vi "kloehn V6 - Parse Pesponse.vi"(8 "error in":errorcluster, 11 "Response String":string) -> (0 "error out":errorcluster, 2 "Status":enum16{"Ready", "Busy"}(ring), 3 "Response String":string)   [LabVIEW 2010]
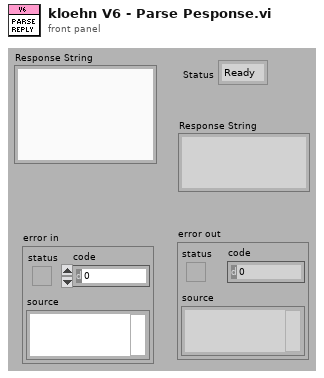
[diagram p1: front panel]
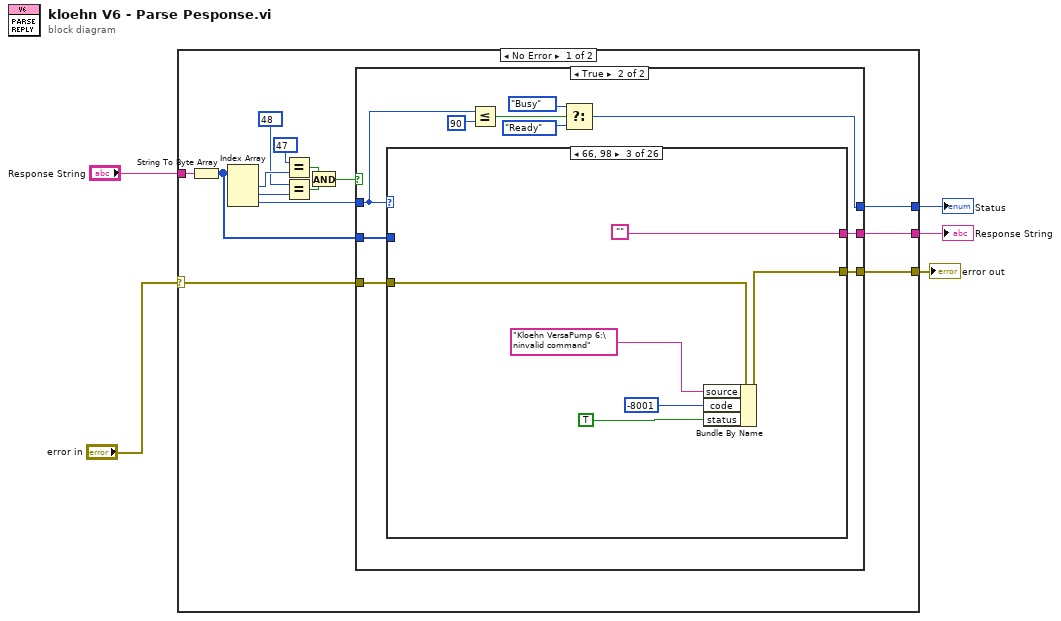
[diagram p0: block diagram]
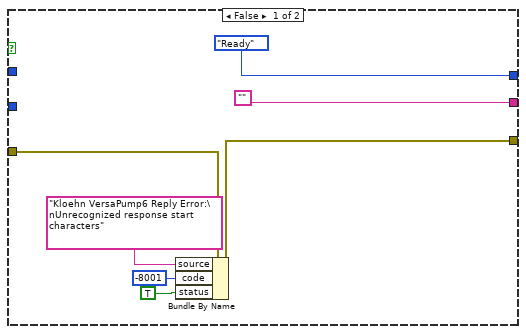
[diagram p2: hidden frame]
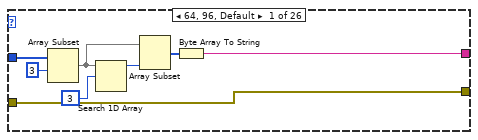
[diagram p3: hidden frame]
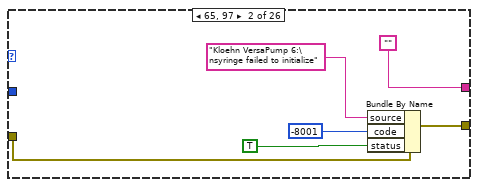
[diagram p4: hidden frame]
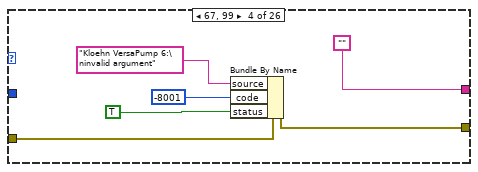
[diagram p5: hidden frame]
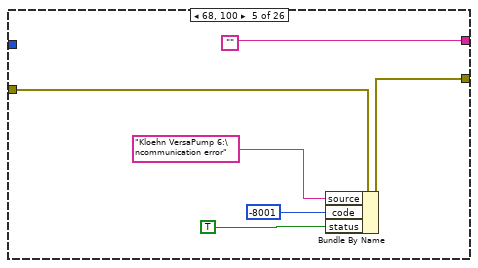
[diagram p6: hidden frame]
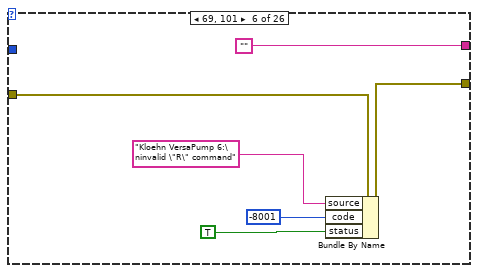
[diagram p7: hidden frame]
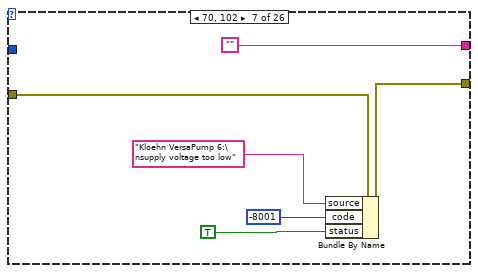
[diagram p8: hidden frame]
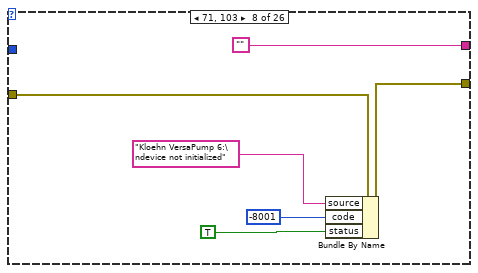
[diagram p9: hidden frame]
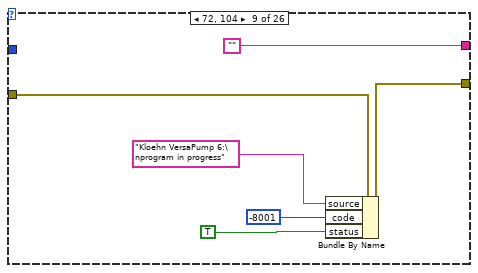
[diagram p10: hidden frame]
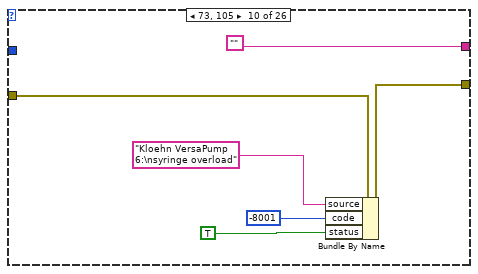
[diagram p11: hidden frame]
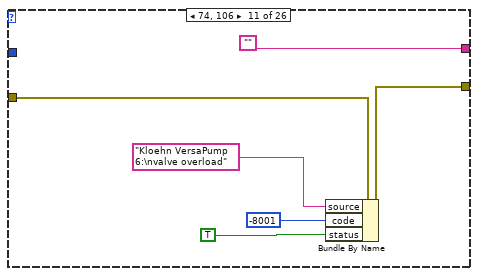
[diagram p12: hidden frame]
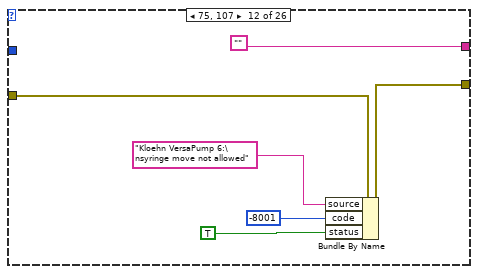
[diagram p13: hidden frame]
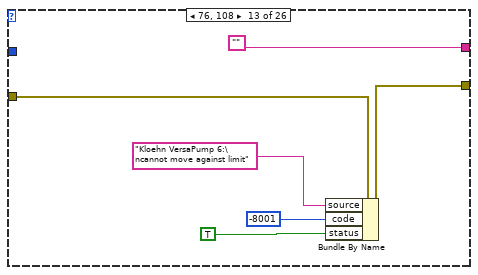
[diagram p14: hidden frame]
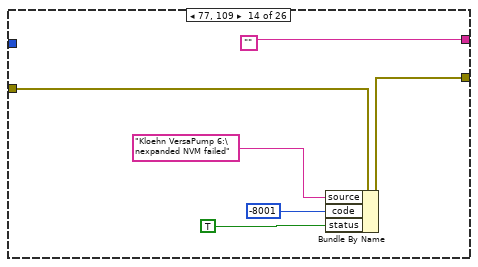
[diagram p15: hidden frame]
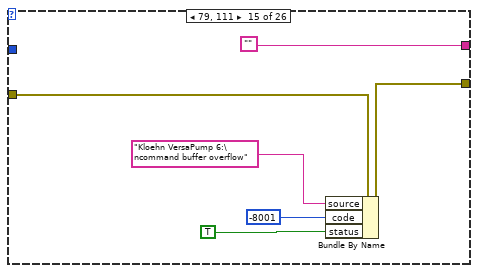
[diagram p16: hidden frame]
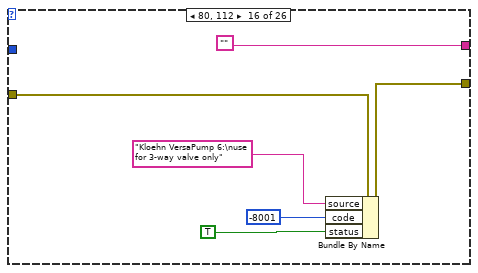
[diagram p17: hidden frame]
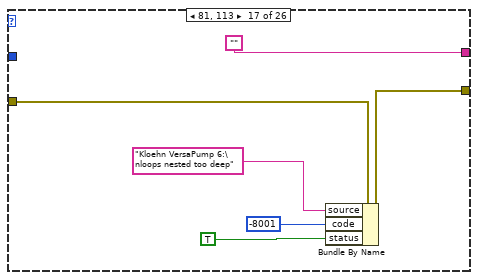
[diagram p18: hidden frame]
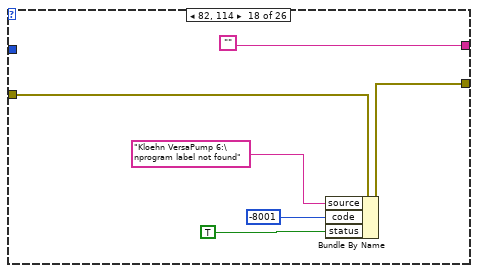
[diagram p19: hidden frame]
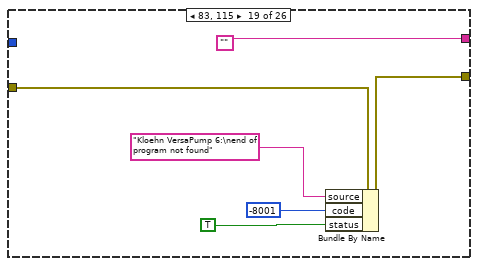
[diagram p20: hidden frame]
diagram:
  n1 = case shown="No Error" "error in" {
    selector: "error in" -> [w11 w197]
    tunnel: "Response String" -> [w19 _]
    tunnel: [w10 w197] -> w3
    tunnel: [w8 enum16{"Ready", "Busy"}."Busy" ("Status")] -> w2
    tunnel: [w6 ""] -> w1
    frame No Error {
      n2 = String To Byte Array(string=w19) -> (unsigned byte array=w7:u8[])
      n3 = Index Array(array=w7) -> (element #1=w18:u8, element #2=w16:u8, element #3=w9:u8)  [unwired: 3 in]
      n4 = Equal?(x=u8 47, y=w18) -> (x = y?=w14:bool)
      n5 = Equal?(x=u8 48, y=w16) -> (x = y?=w13:bool)
      n6 = And(x=w14, y=w13) -> (x .and. y?=w12:bool)
      n7 = case shown="True" w12 {
        tunnel: w11 -> [w26 w36]
        tunnel: [w25 w35] -> w10
        tunnel: w9 -> [_ w30]
        tunnel: [enum16{"Ready", "Busy"}."Ready" ("Status") w29] -> w8
        tunnel: w7 -> [_ w28]
        tunnel: ["" w27] -> w6
        frame False {
          n8 = Bundle By Name(cluster=w26, "source"="Kloehn VersaPump6 Reply Error:\nUnrecognized response start characters", "code"=-8001, "status"=TRUE) -> (w25:errorcluster)
        }
        frame True {
          n9 = case shown="66, 98" w30 {
            tunnel: w36 -> [w44 w50 w56 w62 w68 w74 w80 w86 w92 w98 w104 w110 w116 w122 w128 w134 w140 w146 w152 w158 w164 w170 w176 w182 w188 w194]
            tunnel: [w44 w49 w55 w61 w67 w73 w79 w85 w91 w97 w103 w109 w115 w121 w127 w133 w139 w145 w151 w157 w163 w169 w175 w181 w187 w193] -> w35
            tunnel: w28 -> [w43 _ _ _ _ _ _ _ _ _ _ _ _ _ _ _ _ _ _ _ _ _ _ _ _ _]
            tunnel: [w37 "" "" "" "" "" "" "" "" "" "" "" "" "" "" "" "" "" "" "" "" "" "" "" "" ""] -> w27
            frame 64, 96, Default {
              n10 = Array Subset(array=w43, index=3) -> (w40:u8[])  [unwired: 1 in]
              n11 = Search 1D Array(1D array=w40, element=u8 3 ("index")) -> (index of element=w38:i32)  [unwired: 1 in]
              n12 = Array Subset(array=w40, length=w38) -> (w39:u8[])  [unwired: 1 in]
              n13 = Byte Array To String(unsigned byte array=w39) -> (string=w37:string)
            }
            frame 65, 97 {
              n14 = Bundle By Name(cluster=w50, "source"="Kloehn VersaPump 6:\nsyringe failed to initialize", "code"=-8001, "status"=TRUE) -> (w49:errorcluster)
            }
            frame 66, 98 {
              n15 = Bundle By Name(cluster=w56, "source"="Kloehn VersaPump 6:\ninvalid command", "code"=-8001, "status"=TRUE) -> (w55:errorcluster)
            }
            frame 67, 99 {
              n16 = Bundle By Name(cluster=w62, "source"="Kloehn VersaPump 6:\ninvalid argument", "code"=-8001, "status"=TRUE) -> (w61:errorcluster)
            }
            frame 68, 100 {
              n17 = Bundle By Name(cluster=w68, "source"="Kloehn VersaPump 6:\ncommunication error", "code"=-8001, "status"=TRUE) -> (w67:errorcluster)
            }
            frame 69, 101 {
              n18 = Bundle By Name(cluster=w74, "source"="Kloehn VersaPump 6:\ninvalid \"R\" command", "code"=-8001, "status"=TRUE) -> (w73:errorcluster)
            }
            frame 70, 102 {
              n19 = Bundle By Name(cluster=w80, "source"="Kloehn VersaPump 6:\nsupply voltage too low", "code"=-8001, "status"=TRUE) -> (w79:errorcluster)
            }
            frame 71, 103 {
              n20 = Bundle By Name(cluster=w86, "source"="Kloehn VersaPump 6:\ndevice not initialized", "code"=-8001, "status"=TRUE) -> (w85:errorcluster)
            }
            frame 72, 104 {
              n21 = Bundle By Name(cluster=w92, "source"="Kloehn VersaPump 6:\nprogram in progress", "code"=-8001, "status"=TRUE) -> (w91:errorcluster)
            }
            frame 73, 105 {
              n22 = Bundle By Name(cluster=w98, "source"="Kloehn VersaPump 6:\nsyringe overload", "code"=-8001, "status"=TRUE) -> (w97:errorcluster)
            }
            frame 74, 106 {
              n23 = Bundle By Name(cluster=w104, "source"="Kloehn VersaPump 6:\nvalve overload", "code"=-8001, "status"=TRUE) -> (w103:errorcluster)
            }
            frame 75, 107 {
              n24 = Bundle By Name(cluster=w110, "source"="Kloehn VersaPump 6:\nsyringe move not allowed", "code"=-8001, "status"=TRUE) -> (w109:errorcluster)
            }
            frame 76, 108 {
              n25 = Bundle By Name(cluster=w116, "source"="Kloehn VersaPump 6:\ncannot move against limit", "code"=-8001, "status"=TRUE) -> (w115:errorcluster)
            }
            frame 77, 109 {
              n26 = Bundle By Name(cluster=w122, "source"="Kloehn VersaPump 6:\nexpanded NVM failed", "code"=-8001, "status"=TRUE) -> (w121:errorcluster)
            }
            frame 79, 111 {
              n27 = Bundle By Name(cluster=w128, "source"="Kloehn VersaPump 6:\ncommand buffer overflow", "code"=-8001, "status"=TRUE) -> (w127:errorcluster)
            }
            frame 80, 112 {
              n28 = Bundle By Name(cluster=w134, "source"="Kloehn VersaPump 6:\nuse for 3-way valve only", "code"=-8001, "status"=TRUE) -> (w133:errorcluster)
            }
            frame 81, 113 {
              n29 = Bundle By Name(cluster=w140, "source"="Kloehn VersaPump 6:\nloops nested too deep", "code"=-8001, "status"=TRUE) -> (w139:errorcluster)
            }
            frame 82, 114 {
              n30 = Bundle By Name(cluster=w146, "source"="Kloehn VersaPump 6:\nprogram label not found", "code"=-8001, "status"=TRUE) -> (w145:errorcluster)
            }
            frame 83, 115 {
              n31 = Bundle By Name(cluster=w152, "source"="Kloehn VersaPump 6:\nend of program not found", "code"=-8001, "status"=TRUE) -> (w151:errorcluster)
            }
            frame 84, 116 {
              n32 = Bundle By Name(cluster=w158, "source"="Kloehn VersaPump 6:\nout of program space", "code"=-8001, "status"=TRUE) -> (w157:errorcluster)
            }
            frame 85, 117 {
              n33 = Bundle By Name(cluster=w164, "source"="Kloehn VersaPump 6:\nHOME not set", "code"=-8001, "status"=TRUE) -> (w163:errorcluster)
            }
            frame 86, 118 {
              n34 = Bundle By Name(cluster=w170, "source"="Kloehn VersaPump 6:\ntoo many program calls", "code"=-8001, "status"=TRUE) -> (w169:errorcluster)
            }
            frame 87, 119 {
              n35 = Bundle By Name(cluster=w176, "source"="Kloehn VersaPump 6:\nprogram not found", "code"=-8001, "status"=TRUE) -> (w175:errorcluster)
            }
            frame 88, 120 {
              n36 = Bundle By Name(cluster=w182, "source"="Kloehn VersaPump 6:\nvalve position error", "code"=-8001, "status"=TRUE) -> (w181:errorcluster)
            }
            frame 89, 121 {
              n37 = Bundle By Name(cluster=w188, "source"="Kloehn VersaPump 6:\nsyringe position corrupted", "code"=-8001, "status"=TRUE) -> (w187:errorcluster)
            }
            frame 90, 122 {
              n38 = Bundle By Name(cluster=w194, "source"="Kloehn VersaPump 6:\nsyringe may go past home", "code"=-8001, "status"=TRUE) -> (w193:errorcluster)
            }
          }
          n39 = Less Or Equal?(x=w30, y=u8 90) -> (x <= y?=w32:bool)
          n40 = Select(t=enum16{"Ready", "Busy"}."Busy" ("Status"), s=w32, f=enum16{"Ready", "Busy"}."Ready" ("Status")) -> (s? t:f=w29:enum16{"Ready", "Busy"})
        }
      }
    }
    frame Error {
    }
  }
  "error out" <- w3
  "Status" <- w2
  "Response String" <- w1
